vi "WPI_CameraRead MJPGString.vi"(8 "error in":errorcluster, 9 "fps":i32=30, 10 "Operation":enum16{"Read", "Reopen", "Close"}(ring), 11 "address":string="10.te.am.11") -> (0 "error out":errorcluster, 3 "Raw Image Data":string)   [LabVIEW 2017]
doc: "This VI starts an mjpg stream with the Axis camera at <b>address</b>, decodes the buffer, and places it into the provided <b>image</b>. It is also supports the <b>operation</b> of reopening the stream when <b>camera settings</b> have changed, and the <b>operation</b> of closing the stream.\nUse this VI as an alternative to WPI>>Get Image from Controller. This VI is used for a public camera, Get... is for a cRIO private camera.\n\nThis software is licensed. Open the labview\\readme\\WPI Robotics Library Open Source License.txt file for more information."
uses:
  <resource>/objmgr/LVODE.rc
  <vilib>/robotics/Simulator/NI_Robotics_Simulator.lvlib
panel:
  out "Simulated Camera":refnum<vi>(3d-picture)
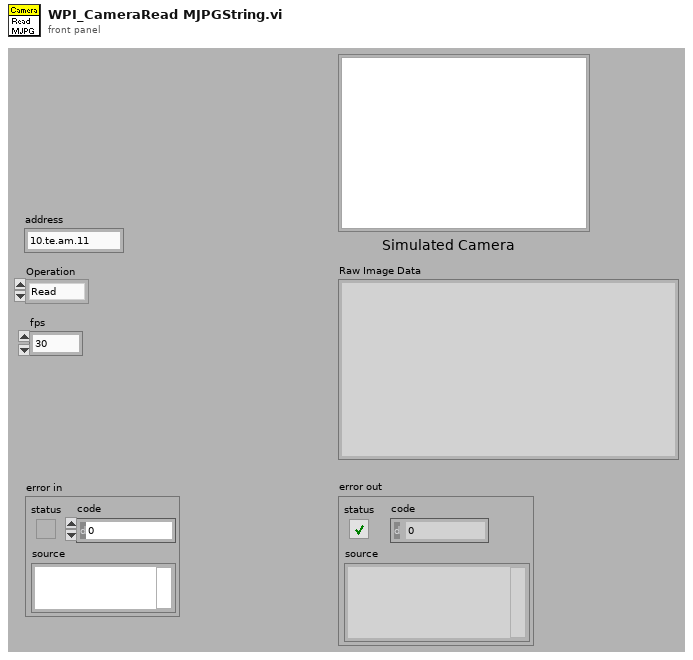
[diagram p1: front panel]
types:
  T1 = cluster{"Position[0]":sgl, "Position[1]":sgl, "Position[2]":sgl}
  T2 = cluster{"Target[0]":sgl, "Target[1]":sgl, "Target[2]":sgl}
  T3 = cluster{"UpDirection[0]":sgl, "UpDirection[1]":sgl, "UpDirection[2]":sgl}
  T4 = typedef "imagedata.ctl" = cluster{"image type":i32, "image depth":i32, "image":u8[], "mask":u8[], "colors":u32[], "Rectangle":cluster{"left":i16, "top":i16, "right":i16, "bottom":i16}}
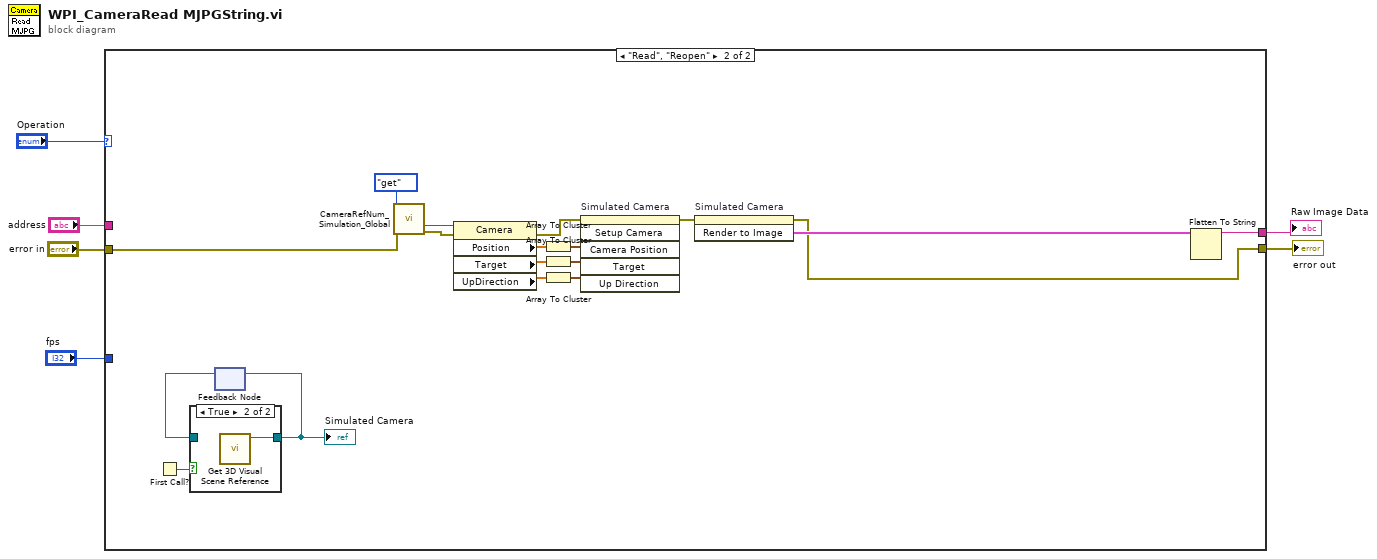
[diagram p0: block diagram]
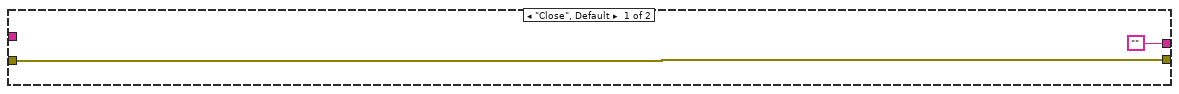
[diagram p2: hidden frame]
diagram:
  n1 = case shown="\"Read\", \"Reopen\"" "Operation" {
    tunnel: "error in" -> [w7 w11]
    tunnel: "address" -> [_ _]
    tunnel: [w7 w9] -> w4
    tunnel: ["" w26] -> w2
    tunnel: "fps" -> [_ _]
    frame "Close", Default {
    }
    frame "Read", "Reopen" {
      n2 = First Call?() -> (First Call?: T/F=w23:bool)
      n3 = feedback #1() -> (w25:refnum<vi>)  [unwired: 1 in]
      n4 = case shown="True" w23 {
        tunnel: [w27 w28] -> w24
        tunnel: w25 -> [w27 _]
        frame False {
        }
        frame True {
          n5 = call <vilib>:"Get 3D Visual Scene Reference.vi"() -> ("scene ref"=w28:refnum<vi>)  [unwired: 10 in, 1 out]
        }
      }
      "Simulated Camera" <- w24
      n6 = feedback-in #1(w24) -> ()
      n7 = call <vilib>:"CameraRefNum_Simulation_Global.vi"("menu"=enum16{"set", "get", "delete"}."get", "error in (no error)"=w11) -> ("Axis M1011 Get"=w14:refnum<k20>, "error out"=w13:errorcluster)  [unwired: 12 in]
      n8 = property class="Camera"(reference=w14, error in=w13) -> (error out=w22:errorcluster, "Position"=w16:sgl[], "Target"=w17:sgl[], "UpDirection"=w18:sgl[])  [unwired: 1 out]
      n9 = Array To Cluster(array=w16) -> (cluster=w19:T1)
      n10 = Array To Cluster(array=w17) -> (cluster=w20:T2)
      n11 = Array To Cluster(array=w18) -> (cluster=w21:T3)
      n12 = invoke on="Simulated Camera" class="SceneGraphDisp (strict)" method="Setup Camera"(error in=w22, "Camera Position"=w19, "Target"=w20, "Up Direction"=w21) -> (error out=w15:errorcluster)  [unwired: 2 in, 5 out]
      n13 = invoke on="Simulated Camera" class="SceneGraphDisp (strict)" method="Render to Image"(error in=w15) -> (error out=w9:errorcluster, "Get Image"=w10:T4)  [unwired: 2 in, 1 out]
      n14 = Flatten To String(anything=w10) -> (data string=w26:string)  [unwired: 3 in, 2 out]
    }
  }
  "error out" <- w4
  "Raw Image Data" <- w2
